vi "Get FPGA Ref.vi"(8 "error in (no error)":errorcluster, 11 "Actor In":refnum<class "Actor.lvclass">) -> (0 "error out":errorcluster, 2 "FPGA Ref":T1, 3 "Actor Out":refnum<class "Actor.lvclass">)   [LabVIEW 2017, in "Controller.lvlib" / "gController.lvclass"]
uses:
  gController.lvclass
  FPGA Ref.ctl
  <vilib>/ActorFramework/Actor/Actor.lvclass
  C:/Program Files (x86)/National Instruments/LabVIEW 2017/vi.lib/ActorFramework/Actor/Actor.lvclass
  gController.lvclass/gController.ctl
  Session/Raw FPGA/FPGA Session.lvclass/FPGA Session.ctl
  Read FPGA Session.vi
  Session/Raw FPGA/Read FPGA Ref.vi
  Session/Raw FPGA/FPGA Session.lvclass
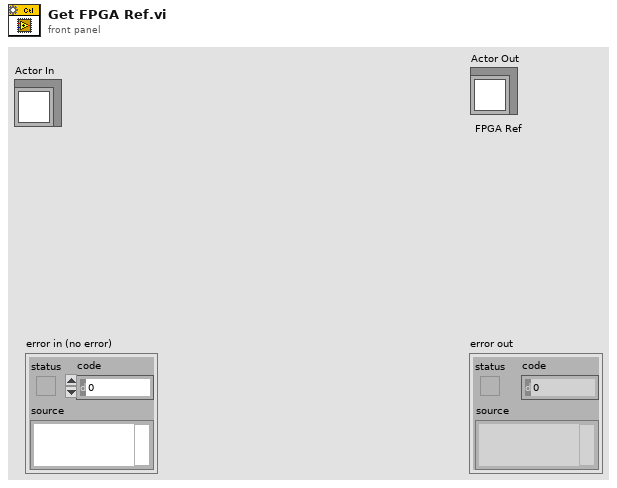
[diagram p1: front panel]
types:
  T1 = typedef "FPGA Ref.ctl" = refnum<k20>
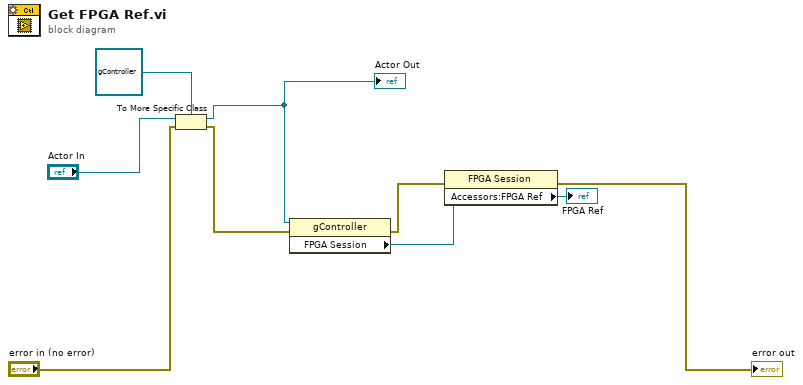
[diagram p0: block diagram]
diagram:
  n1 = To More Specific Class(target class=refnum<class "gController.lvclass"> refnum ("Controller.lvlib:gController"), reference="Actor In", error in="error in (no error)") -> (specific class reference=w1:refnum<class "gController.lvclass">, error out=w5:errorcluster)
  "Actor Out" <- w1
  n2 = property class="gController"(reference=w1, error in=w5) -> (error out=w4:errorcluster, "FPGA Session"=w9:refnum<data-value>)  [unwired: 1 out]
  n3 = property class="FPGA Session"(reference=w9, error in=w4) -> (error out=→"error out":errorcluster, "Accessors:FPGA Ref"=→"FPGA Ref":T1)  [unwired: 1 out]
